vi "MFCRead.vi"(8 "Error In":errorcluster, 11 "Sierra M100 In":refnum<visa-resource-name>) -> (0 "Error Out":errorcluster, 2 "Flow Rate":dbl, 3 "Sierra M100 Out":refnum<visa-resource-name>)   [LabVIEW 2012]
uses:
  libs/Sierra-M100/Sierra-M100.lvlib
  libs/LV-Utilities/LV-Utilities.lvlib
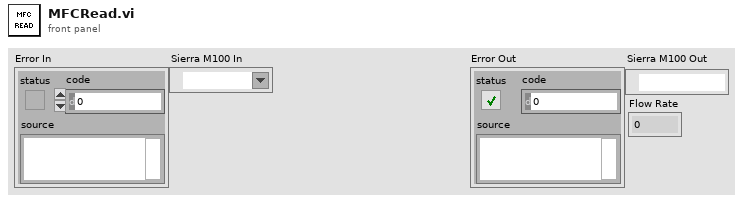
[diagram p1: front panel]
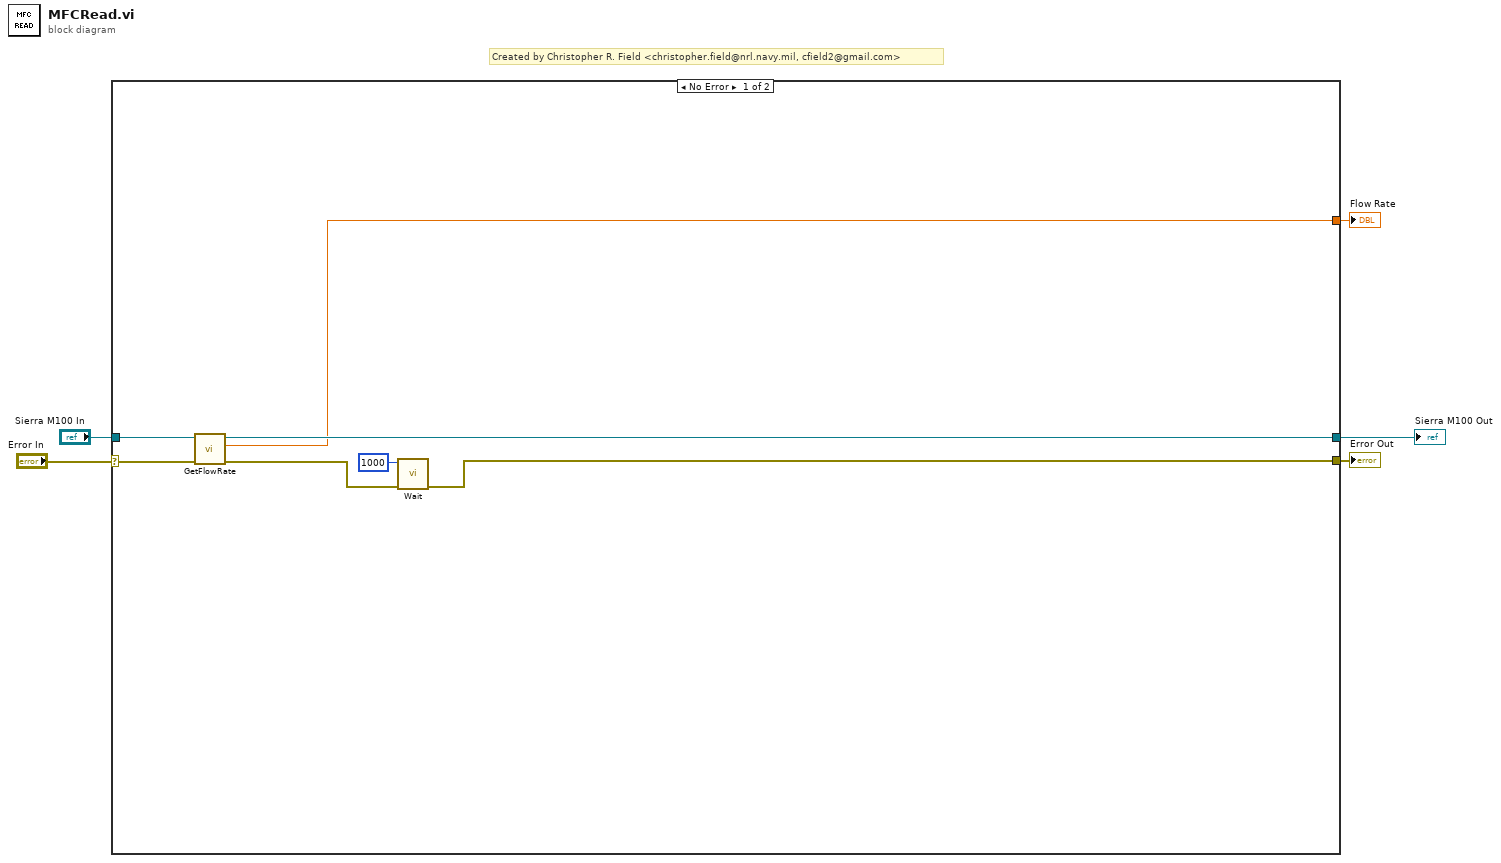
[diagram p0: block diagram]
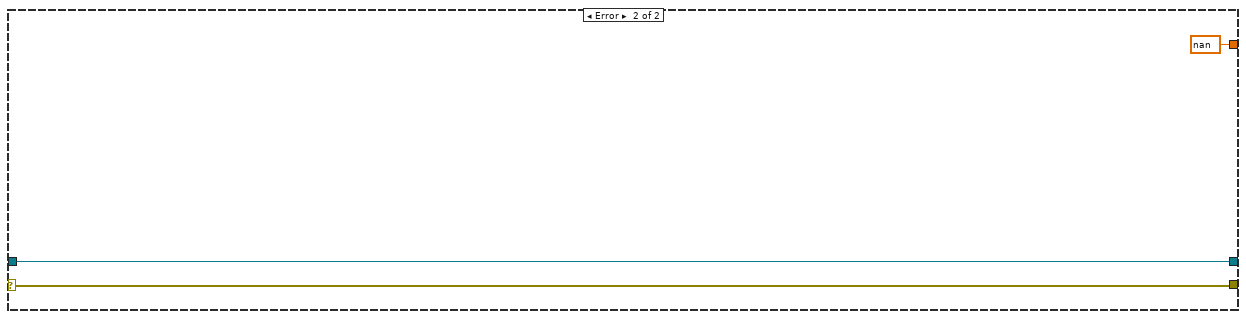
[diagram p2: hidden frame]
diagram:
  # "Created by Christopher R. Field <christopher.field@nrl.navy.mil, cfield2@gmail.com>"
  n1 = case shown="No Error" "Error In" {
    selector: "Error In" -> [w10 w13]
    tunnel: [w9 w13] -> w4
    tunnel: [w8 w14] -> w3
    tunnel: "Sierra M100 In" -> [w7 w14]
    tunnel: [w6 nan ("Flow Rate")] -> w1
    frame No Error {
      n2 = call "GetFlowRate.vi"("Error In"=w10, "Sierra M100 In"=w7) -> ("Error Out"=w12:errorcluster, "Flow Rate"=w6:dbl, "Sierra M100 Out"=w8:refnum<visa-resource-name>)  [unwired: 6 in, 1 out]
      n3 = call "Wait.vi"("Error In"=w12, "Wait Time (msec)"=u32 1000) -> ("Error Out"=w9:errorcluster)  [unwired: 9 in]
    }
    frame Error {
    }
  }
  "Error Out" <- w4
  "Sierra M100 Out" <- w3
  "Flow Rate" <- w1
